vi "NOx_Example_RT.vi"() -> ()   [LabVIEW 2011]
uses:
  <vilib>/Platform/TimedLoop/XDataNode/XDataNode.xnode
  <vilib>/Platform/TimedLoop/XDataNode/nitl_modes.ctl
  <vilib>/Platform/TimedLoop/XDataNode/XDNodeRunTimeDep.lvlib
  <vilib>/Platform/TimedLoop/XDataNode/wakeup.ctl
  <vilib>/Platform/TimedLoop/XDataNode/timing_clust.ctl
  <vilib>/rvi/interface/nirviCloseFPGA/nirviCloseFPGA.xnode
  <vilib>/rvi/interface/nirviOpenFPGA/nirviOpenFPGA.xnode
  W:/Data/Drivven/Products/Device Drivers/.LabVIEW 2010/Examples/Device Drivers/NOx - RevA/NOx_Example_FPGA.vi
  <vilib>/rvi/interface/nirviReadWriteControl/nirviReadWriteControl.xnode
  <vilib>/rvi/errors/niLvFpgaMergeErrorWithErrorCode.vi
  <vilib>/rvi/errors/niLvFpgaAdjustHostInterfaceError.vi
  <vilib>/FPGAPlugInAG/cRIO-9103/niLvFpga_Close_cRIO-9103.vi
panel:
  out "NOxSensorData 2":T1={"NOx (ppm)"=0.0, "O2 (%)"=0.0, "Sensor Supply Status"=3, "Sensor Temperature Status"=12, "NOx Signal Status"=48, "O2 Signal Status"=192, "Heater Mode Status"=96, "Heater Circuit Status"=31, "NOx Circuit Status"=31, "O2 Circuit Status"=31, "NOx Sensor Module Present"=FALSE} {"Heater Mode Status" items=["AUTO MODE"=0, "HEATUP SLOPE 3 OR 4"=32, "HEATUP SLOPE 1 OR 2"=64, "HEATER OFF / PREHEAT"=96]; "O2 Circuit Status" items=["OPEN WIRE"=3, "SHORT CIRCUIT"=5, "NO ERROR"=31]; "NOx Circuit Status" items=["OPEN WIRE"=3, "SHORT CIRCUIT"=5, "NO ERROR"=31]; "Heater Circuit Status" items=["OPEN WIRE"=3, "SHORT CIRCUIT"=5, "NO ERROR"=31]; "Sensor Temperature Status" items=["NOT AT TEMPERATURE"=0, "AT TEMPERATURE"=4, "ERROR"=8, "NOT AVAILABLE"=12]; "O2 Signal Status" items=["NOT VALID"=0, "VALID"=64, "ERROR"=128, "NOT AVAILABLE"=192]; "NOx Signal Status" items=["NOT VALID"=0, "VALID"=16, "ERROR"=32, "NOT AVAILABLE"=48]; "Sensor Supply Status" items=["NOT IN RANGE", "SUPPLY IN RANGE", "ERROR", "NOT AVAILABLE"]}
  out "NOxSensorData 1":T1={"NOx (ppm)"=0.0, "O2 (%)"=0.0, "Sensor Supply Status"=3, "Sensor Temperature Status"=12, "NOx Signal Status"=48, "O2 Signal Status"=192, "Heater Mode Status"=96, "Heater Circuit Status"=31, "NOx Circuit Status"=31, "O2 Circuit Status"=31, "NOx Sensor Module Present"=FALSE} {"Heater Mode Status" items=["AUTO MODE"=0, "HEATUP SLOPE 3 OR 4"=32, "HEATUP SLOPE 1 OR 2"=64, "HEATER OFF / PREHEAT"=96]; "O2 Circuit Status" items=["OPEN WIRE"=3, "SHORT CIRCUIT"=5, "NO ERROR"=31]; "NOx Circuit Status" items=["OPEN WIRE"=3, "SHORT CIRCUIT"=5, "NO ERROR"=31]; "Heater Circuit Status" items=["OPEN WIRE"=3, "SHORT CIRCUIT"=5, "NO ERROR"=31]; "Sensor Temperature Status" items=["NOT AT TEMPERATURE"=0, "AT TEMPERATURE"=4, "ERROR"=8, "NOT AVAILABLE"=12]; "O2 Signal Status" items=["NOT VALID"=0, "VALID"=64, "ERROR"=128, "NOT AVAILABLE"=192]; "NOx Signal Status" items=["NOT VALID"=0, "VALID"=16, "ERROR"=32, "NOT AVAILABLE"=48]; "Sensor Supply Status" items=["NOT IN RANGE", "SUPPLY IN RANGE", "ERROR", "NOT AVAILABLE"]}
  out "Iteration Duration":u64
  in  "RxID 2":u32=418385489 format="%08x"
  in  "Sensor 2 Enable":bool
  in  "stop":bool
  out "FPGA Status":errorcluster
  in  "Sensor 1 Enable":bool
  in  "RxID 1":u32=418385746 format="%08x"
  in  "TxID":u32=419356416 format="%08x"
  in  "CAN Restart":bool
  out "Sensor Results Chart":T2(graph)
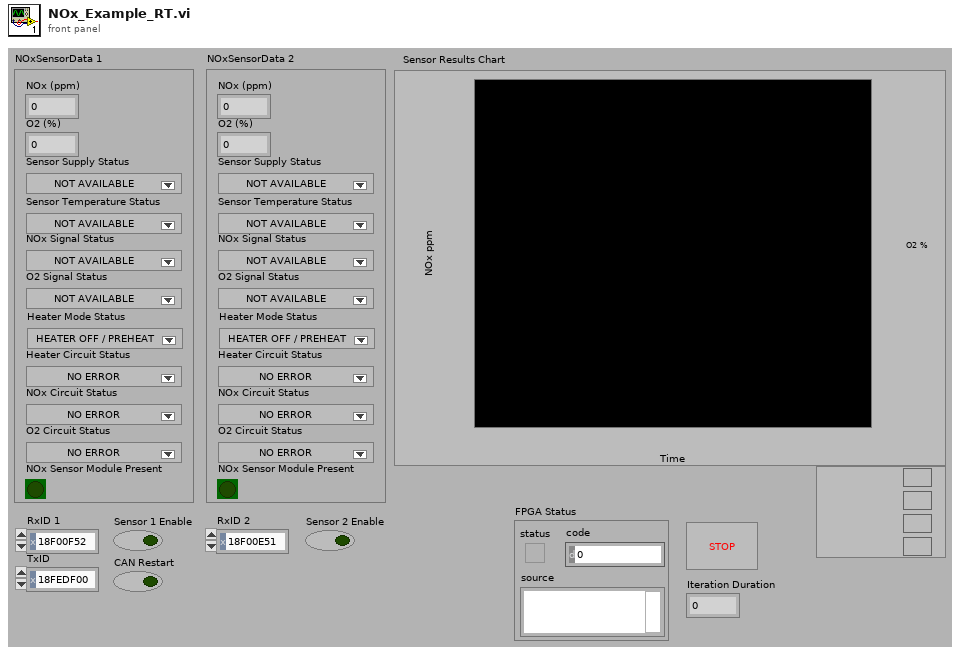
[diagram p1: front panel]
types:
  T1 = cluster{"NOx (ppm)":sgl, "O2 (%)":sgl, "Sensor Supply Status":u8, "Sensor Temperature Status":u8, "NOx Signal Status":u8, "O2 Signal Status":u8, "Heater Mode Status":u8, "Heater Circuit Status":u8, "NOx Circuit Status":u8, "O2 Circuit Status":u8, "NOx Sensor Module Present":bool}
  T2 = cluster{"NOx (ppm)":sgl, "O2 (%)":sgl, "NOx (ppm)":sgl, "O2 (%)":sgl}
  T3 = typedef "XDNodeRunTimeDep.lvlib/timing_clust.ctl" = cluster{"Expected End [f-1]":u64, "Actual End [f-1]":u64, "Finished Late? [f-1]":bool, "Expected End [i-1]":u64, "Actual End [i-1]":u64, "Finished Late? [i-1]":bool, "Expected Start [i]":u64, "Actual Start [i]":u64, "Expected Start [f]":u64, "Actual Start [f]":u64, "Source Name":string, "Structure Name":string, "Period":i64, "Deadline":i64, "Offset":i64, "Start":i64, "Priority":i32, "Timeout":i32, "Mode":T4, "Wakeup Reason":T5, "Error":errorcluster, "Source Type":string, "Secondary Source Type":string, "Global End Time":u64, "Global Start Time":u64, "Frame Duration":u64, "Iteration Duration":u64, "Assigned CPU":i32, "I/O Scan Engine Mode":u32}
  T4 = typedef "XDNodeRunTimeDep.lvlib/nitl_modes.ctl" = enum32{"No Change", "Process missed periods, maintain original phase", "Discard missed periods, maintain original phase", "Process missed periods, ignore original phase", "Discard missed periods, ignore original phase"}
  T5 = typedef "XDNodeRunTimeDep.lvlib/wakeup.ctl" = enum32{"Normal", "Aborted", "Asynchronous wakeup", "Timing source error", "Timed loop error", "Timeout"}
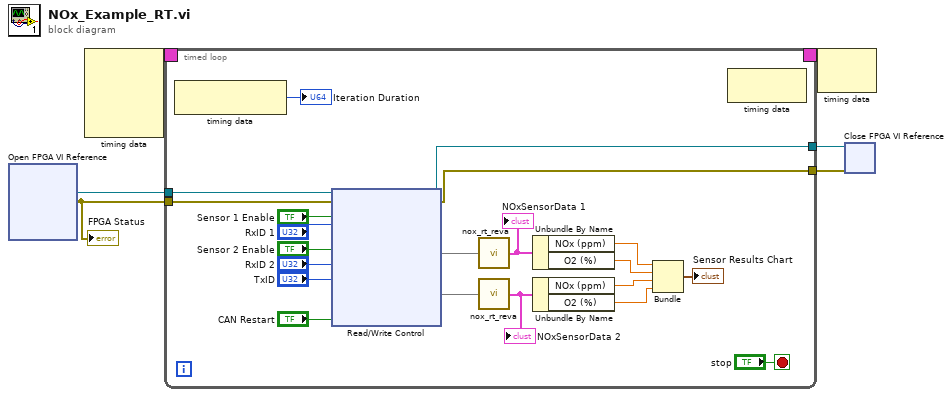
[diagram p0: block diagram]
diagram:
  n1 = xnode "Open FPGA VI Reference"() -> ("FPGA VI Reference Out"=w2:refnum<k20>, "error out"=w1:errorcluster)  [unwired: 2 in]
  "FPGA Status" <- w1
  n2 = node-c288() -> (w6:T3)  [unwired: 4 out]
  n3 = timed-loop {
    timing: w6 -> [_]
    timing-out: [_] -> w5
    tunnel: w2 -> [w18]
    tunnel: [w8] -> w4
    tunnel: w1 -> [w17]
    tunnel: [w7] -> w3
    stop <- "stop" stop-if-true
    n4 = node-c288() -> (→"Iteration Duration":i64)  [unwired: 1 out]
    n5 = xnode "Read/Write Control"("FPGA VI Reference In"=w18, "error in"=w17, "Sensor 1 Enable"="Sensor 1 Enable", "RxID 1"="RxID 1", "Sensor 2 Enable"="Sensor 2 Enable", "RxID 2"="RxID 2", "TxID"="TxID", "CAN0 Restart"="CAN Restart") -> ("FPGA VI Reference Out"=w8:refnum<k20>, "error out"=w7:errorcluster, "NOxSensorData 1"=w10, "NOxSensorData 2"=w9)
    n6 = call <vilib>:"nox_rt_reva.vi"("NOxSensorDataFromFPGA"=w10) -> ("NOxSensorData"=w24:T1)
    "NOxSensorData 1" <- w24
    n7 = call <vilib>:"nox_rt_reva.vi"("NOxSensorDataFromFPGA"=w9) -> ("NOxSensorData"=w22:T1)
    "NOxSensorData 2" <- w22
    n8 = Unbundle By Name(w24) -> ("NOx (ppm)"=w26:sgl, "O2 (%)"=w23:sgl)
    n9 = Unbundle By Name(w22) -> ("NOx (ppm)"=w21:sgl, "O2 (%)"=w20:sgl)
    n10 = Bundle("NOx (ppm)"=w26, "O2 (%)"=w23, "NOx (ppm)"=w21, "O2 (%)"=w20) -> (→"Sensor Results Chart":T2)  [unwired: 1 out]
    n11 = node-c288() -> ()  [unwired: 2 out]
  }
  n12 = node-c288(w5) -> ()  [unwired: 1 out]
  n13 = xnode "Close FPGA VI Reference"("FPGA VI Reference In"=w4, "error in"=w3) -> ()  [unwired: 1 out]
